vi "test Create Default Anchor.vi"(8 "error in (no error)":errorcluster, 11 "TestCase in":refnum<class "AnchorTests.lvclass">) -> (0 "error out":errorcluster, 3 "TestCase out":refnum<class "AnchorTests.lvclass">)   [LabVIEW 2014, in "AnchorTests.lvclass"]
uses:
  AnchorTests.lvclass
  <vilib>/addons/_JKI Toolkits/VI Tester/TestCase.llb/TestCase.lvclass
  SPLAT/Anchor/Anchor.lvclass
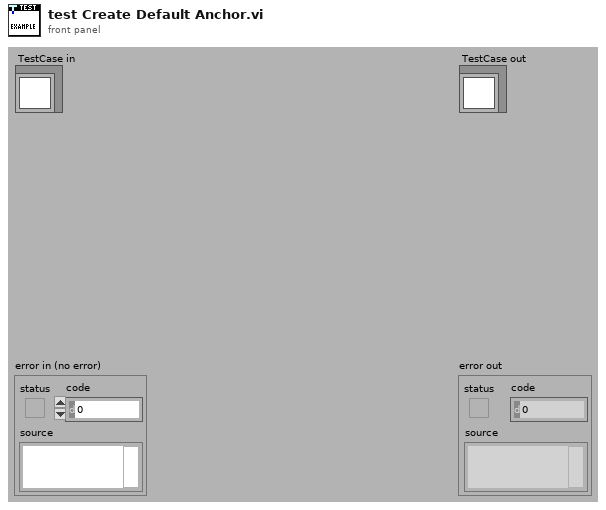
[diagram p1: front panel]
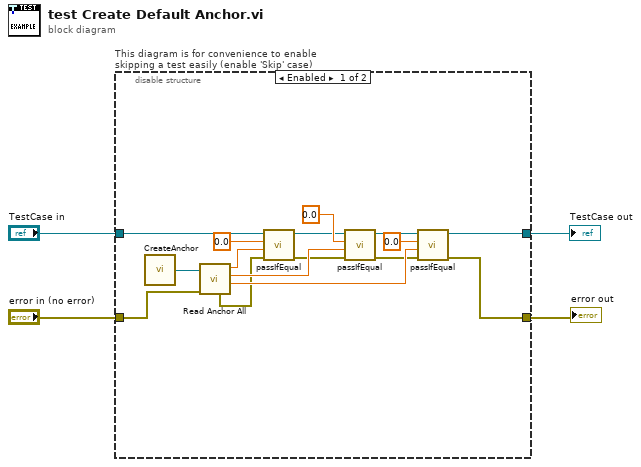
[diagram p0: block diagram]
diagram:
  n1 = disable-structure "This diagram is for convenience to enable skipping a test easily (enable 'Skip' case)" shown="Enabled" {
    disable-tunnel: "TestCase in" -> [w13 w24]
    disable-tunnel: [w10 w22] -> w1
    disable-tunnel: [w5 w23] -> w3
    disable-tunnel: "error in (no error)" -> [w9 w21]
    frame Enabled {
      n2 = call "CreateAnchor.vi"() -> ("Anchor Out"=w20:refnum<class "Anchor.lvclass">)  [unwired: 3 in]
      n3 = call "Read Anchor All.vi"("error in (no error)"=w9, "Anchor in"=w20) -> ("AnchorY"=w15:dbl, "AnchorX"=w17:dbl, "AnchorID"=w19:dbl, "error out"=w8:errorcluster)  [unwired: 4 in, 2 out]
      n4 = call-dynamic "passIfEqual.vi"("error in (no error)"=w8, "y"=w19, "x"=0.0, "TestCase in"=w13) -> ("error out"=w7:errorcluster, "TestCase out"=w12:refnum<class "AnchorTests.lvclass">)  [unwired: 6 in]
      n5 = call-dynamic "passIfEqual.vi"("error in (no error)"=w7, "y"=w17, "x"=0.0, "TestCase in"=w12) -> ("error out"=w6:errorcluster, "TestCase out"=w11:refnum<class "AnchorTests.lvclass">)  [unwired: 6 in]
      n6 = call-dynamic "passIfEqual.vi"("error in (no error)"=w6, "y"=w15, "x"=0.0, "TestCase in"=w11) -> ("error out"=w5:errorcluster, "TestCase out"=w10:refnum<class "AnchorTests.lvclass">)  [unwired: 6 in]
    }
    frame Disabled {
      # "skip test result while test is under development"
      n7 = call <vilib>:"skip.vi"("error in (no error)"=w21, "TestCase in"=w24) -> ("error out"=w23:errorcluster, "TestCase out"=w22:refnum<class "AnchorTests.lvclass">)  [unwired: 8 in]
    }
  }
  "error out" <- w3
  "TestCase out" <- w1
